vi "CloseFont.vi"(8 "No Error":errorcluster, 11 "Font [TTF_Font *]":i64 format="%.0x") -> (0 "error out":errorcluster)   [LabVIEW 2024, in "SDL3.lvlib" / "TTF.lvlib"]
doc: "<B>Summary</B>\nDispose of a previously-created font.\n\n<B>Remarks</B>\nCall this when done with a font. This function will free any resources associated with it. It is safe to call this function on NULL, for example on the result of a failed call to <B>TTF_OpenFont()</B>.\n\nThe font is not valid after being passed to this function. String pointers from functions that return information on this font, such as <B>TTF_GetFontFamilyName()</B> and <B>TTF_GetFontStyleName()</B>, are no longer valid after this call, as well."
uses:
  TTF.lvlib
  Lib/SDL3_ttf.dll
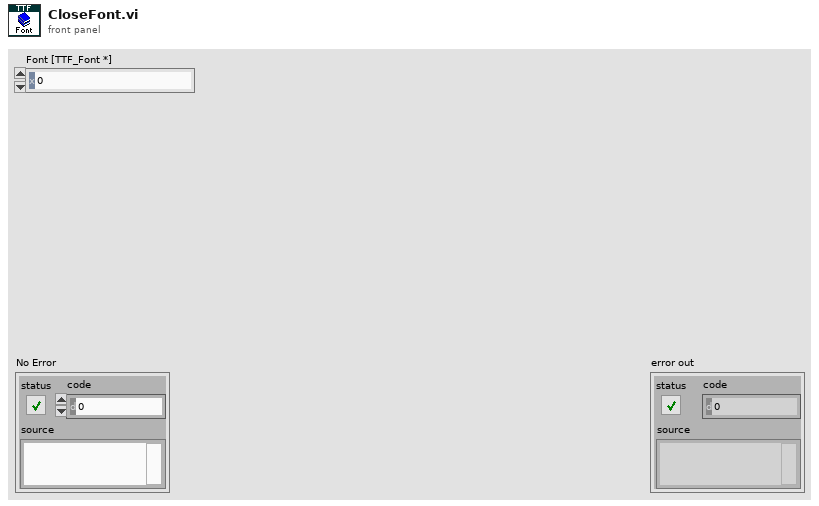
[diagram p1: front panel]
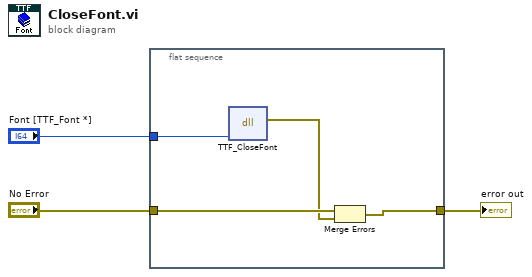
[diagram p0: block diagram]
diagram:
  n1 = flat-sequence {
    tunnel: "No Error" -> [w7]
    tunnel: [w6] -> w2
    tunnel: "Font [TTF_Font *]" -> [w4]
    frame #0 {
      n2 = dll-call lib="C:/Users/Thomas/Documents/Projects/LV-SDL3/Sources/SDL3/Lib/SDL3_ttf.*" fn="TTF_CloseFont"("font"=w4) -> (error out=w5:errorcluster)  [unwired: 5 in, 1 out]
      n3 = Merge Errors(w7, w5) -> (w6:errorcluster)
    }
  }
  "error out" <- w2
